vi "DisplayFilesToMerge_Valise.vi"(6 "Error In":errorcluster, 9 "MergeFileConfigIN":T1) -> (0 "Error Out":errorcluster, 1 "NortekWaveForms":waveform(dbl)[](graph), 2 "HexapodWaveForms":waveform(dbl)[](graph), 3 "QualisysWaveform":waveform(dbl)[](graph), 4 "ValiseWaveform":waveform(dbl)[](graph))   [LabVIEW 2017]
uses:
  DefDeType/MergeFileConfig.ctl
  DefDeType/WhichPath.ctl
panel:
  out "size(s)":i32
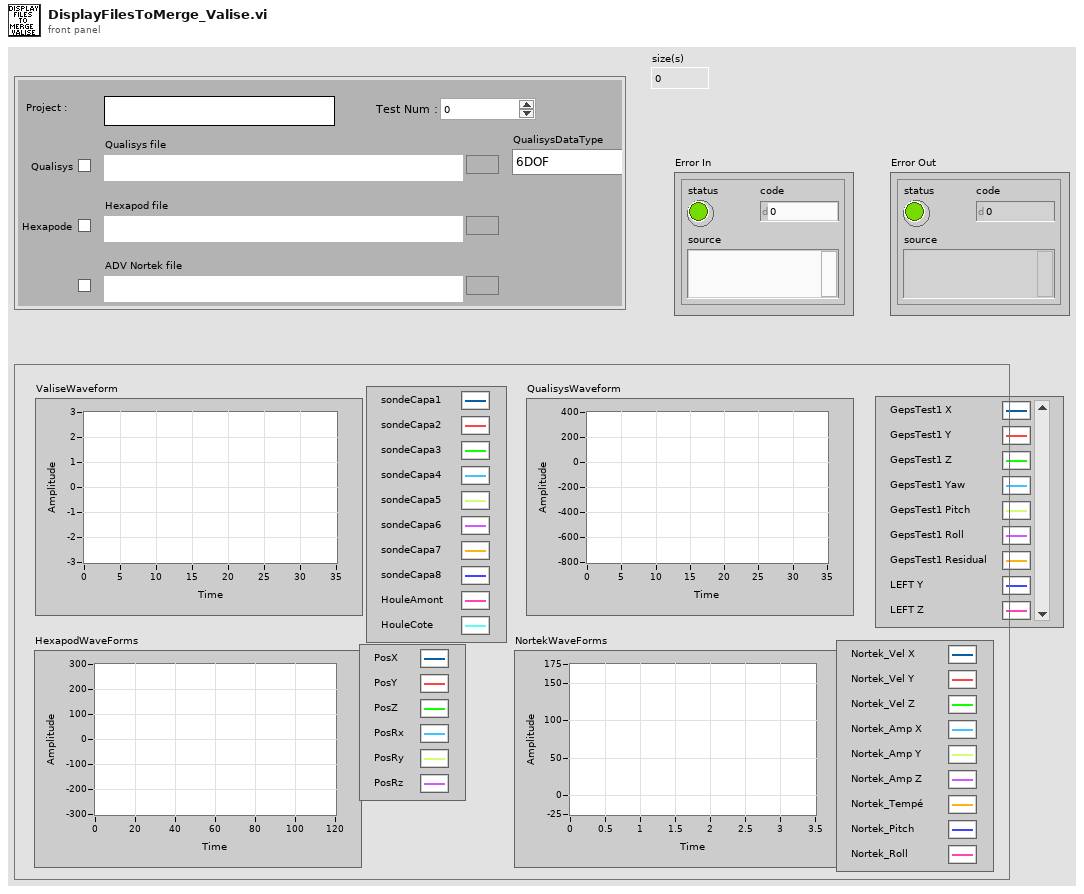
[diagram p1: front panel]
types:
  T1 = typedef "MergeFileConfig.ctl" = cluster{"Test Num : ":u32, "Project :":string, "Qualisys file":path, "Hexapod file":path, "ADV Nortek file":path, "QualisysDataType":enum16{"6DOF", "3DTracking", "6DOF + 3D"}, "Qualisys":bool, "Hexapode":bool, "ADV Nortek":bool}
  T2 = typedef "WhichPath.ctl" = enum16{"DossierProjet", "Config", "Meas", "MeasPCI", "MeasCRIO1", "MeasCRIO2", "MeasQualisys", "MeasHBM", "MeasTDMS", "Fig", "Res"}
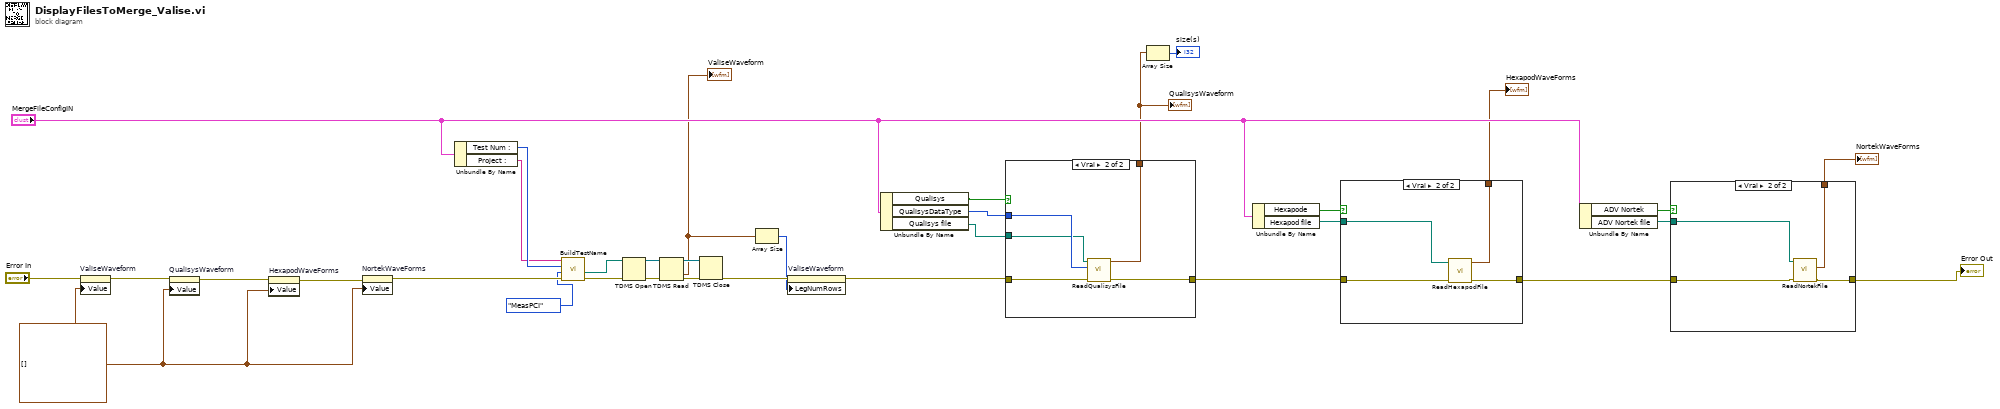
[diagram p0: block diagram]
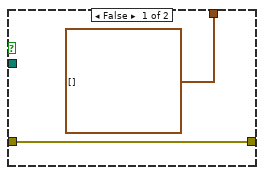
[diagram p2: hidden frame]
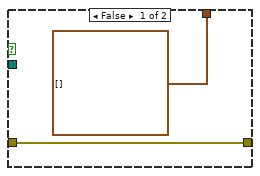
[diagram p3: hidden frame]
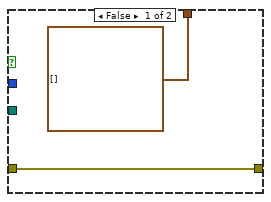
[diagram p4: hidden frame]
diagram:
  w30 = waveform(dbl)[] [] ("QualisysWaveforms")
  n1 = property on="ValiseWaveform" class="GraphWF (strict)"(error in="Error In", "Value"=w30) -> (error out=w33:errorcluster)  [unwired: 1 in, 1 out]
  n2 = property on="QualisysWaveform" class="GraphWF (strict)"(error in=w33, "Value"=w30) -> (error out=w32:errorcluster)  [unwired: 1 in, 1 out]
  n3 = property on="HexapodWaveForms" class="GraphWF (strict)"(error in=w32, "Value"=w30) -> (error out=w31:errorcluster)  [unwired: 1 in, 1 out]
  n4 = property on="NortekWaveForms" class="GraphWF (strict)"(error in=w31, "Value"=w30) -> (error out=w22:errorcluster)  [unwired: 1 in, 1 out]
  n5 = Unbundle By Name("MergeFileConfigIN") -> ("Test Num :"=w27:u32, "Project :"=w18:string)
  n6 = call "BuildTestName.vi"("entrée d'erreur"=w22, "WhichPath?"=WhichPath."MeasPCI", "NextTestNum"=w27, "NomProjet"=w18) -> ("sortie d'erreur"=w29:errorcluster, "cheminProchainFichier"=w28:path)  [unwired: 1 in, 2 out]
  n7 = TDMS Open(8:w29, 11:w28) -> (0:w25:errorcluster, 3:w26:refnum<k34>)  [unwired: 5 in]
  n8 = TDMS Read(0:w26, 11:w25) -> (4:w24:refnum<k34>, 10:w4:waveform(dbl)[], 15:w23:errorcluster)  [unwired: 6 in, 3 out]
  "ValiseWaveform" <- w4
  n9 = TDMS Close(8:w23, 11:w24) -> (0:w6:errorcluster)  [unwired: 1 out]
  n10 = Array Size(array=w4) -> (size(s)=w3:i32)
  n11 = property on="ValiseWaveform" class="GraphWF (strict)"(error in=w6, "LegNumRows"=w3) -> (error out=w5:errorcluster)  [unwired: 1 in, 1 out]
  n12 = Unbundle By Name("MergeFileConfigIN") -> ("Qualisys"=w19:bool, "QualisysDataType"=w20:enum16{"6DOF", "3DTracking", "6DOF + 3D"}, "Qualisys file"=w21:path)
  n13 = case shown="Vrai" w19 {
    tunnel: [w36 w41] -> w14
    tunnel: w5 -> [w36 w37]
    tunnel: w20 -> [_ w40]
    tunnel: [waveform(dbl)[] [] ("QualisysWaveforms") w39] -> w2
    tunnel: w21 -> [_ w38]
    frame False {
    }
    frame True {
      n14 = call "ReadQualisysFile.vi"("sortie d'erreur"=w37, "QualisysDataType"=w40, "FichierQualisys"=w38) -> ("error out"=w41:errorcluster, "QualisysWaveforms"=w39:waveform(dbl)[])  [unwired: 3 in]
    }
  }
  "QualisysWaveform" <- w2
  n15 = Array Size(array=w2) -> (size(s)=→"size(s)":i32)
  n16 = Unbundle By Name("MergeFileConfigIN") -> ("Hexapode"=w16:bool, "Hexapod file"=w15:path)
  n17 = case shown="Vrai" w16 {
    tunnel: w14 -> [w43 w44]
    tunnel: [w43 w47] -> w12
    tunnel: [waveform(dbl)[] [] ("QualisysWaveforms") w46] -> w7
    tunnel: w15 -> [_ w45]
    frame False {
    }
    frame True {
      n18 = call "ReadHexapodFile.vi"("error in (not an error)"=w44, "file path (use dialog)"=w45) -> ("error out"=w47:errorcluster, "WaveformsHexapode"=w46:waveform(dbl)[])  [unwired: 4 in]
    }
  }
  "HexapodWaveForms" <- w7
  n19 = Unbundle By Name("MergeFileConfigIN") -> ("ADV Nortek"=w10:bool, "ADV Nortek file"=w13:path)
  n20 = case shown="Vrai" w10 {
    tunnel: [w48 w53] -> w9
    tunnel: [waveform(dbl)[] [] ("QualisysWaveforms") w52] -> w8
    tunnel: w13 -> [_ w50]
    tunnel: w12 -> [w48 w51]
    frame False {
    }
    frame True {
      n21 = call "ReadNortekFile.vi"("error in"=w51, "FichierNortek"=w50) -> ("error out"=w53:errorcluster, "Nortek WaveForms"=w52:waveform(dbl)[])  [unwired: 4 in]
    }
  }
  "NortekWaveForms" <- w8
  "Error Out" <- w9
